vi "Periodic Tasks.vi"(8 "error in":errorcluster) -> ()   [LabVIEW 2020]
doc: "This VI runs in parallel to other robot code. It can contain as many user-defined periodic loops as you need. These can carry out PID or other sorts of timed response."
uses:
  <vilib>/Rock Robotics/WPI/Utilities/WPI_GetSetVariantRefNum.vi
  Robot Global Data.vi
  <vilib>/Rock Robotics/Network Tables/NT Read String.vi
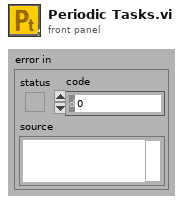
[diagram p1: front panel]
types:
  T1 = typedef "WPI_JoystickDevRef.ctl" = cluster{"Device":T2}
  T2 = typedef "WPI_JoystickDeviceEnum.ctl" = enum16{"USB 0", "USB 1", "USB 2", "USB 3", "USB 4", "USB 5"}
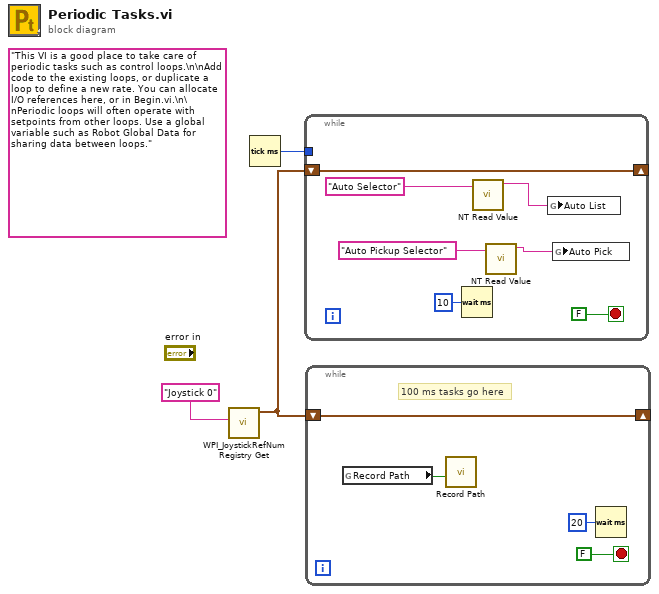
[diagram p0: block diagram]
diagram:
  (unwired) "This VI is a good place to take care of periodic tasks such as control loops.\n\nAdd code to the existing loops, or duplicate a loop to define a new rate. You can allocate I/O references here, or in Begin.vi.\n\nPeriodic loops will often operate with setpoints from other loops. Use a global variable such as Robot Global Data for sharing data between loops."
  n1 = call <vilib>:"WPI_JoystickRefNum Registry Get.vi"("refnum name"="Joystick 0") -> ("JoystickDevRef"=w2:T1)  [unwired: 1 in, 9 out]
  n2 = Tick Count (ms)() -> (millisecond timer value=w1:u32)
  n3 = while {
    shift-right: [w9] -> _
    shift-left: w2 -> [w9]
    tunnel: w1 -> [_]
    stop <- FALSE stop-if-true
    n4 = Wait (ms)(milliseconds to wait=u32 10) -> ()  [unwired: 1 out]
    n5 = call-poly <vilib>:"NT Read Value.vi"("Name"="Auto Selector") -> ("String"=w6:string)  [unwired: 9 in, 1 out]
    n6 = call-poly <vilib>:"NT Read Value.vi"("Name"="Auto Pickup Selector") -> ("String"=w7:string)  [unwired: 9 in, 1 out]
    n7 = global write "Robot Global Data.vi" "Auto List"(w6) -> ()
    n8 = global write "Robot Global Data.vi" "Auto Pick"(w7) -> ()
  }
  n9 = while {
    shift-right: [w12] -> _
    shift-left: w2 -> [w12]
    stop <- FALSE stop-if-true
    # "100 ms tasks go here"
    n10 = global read "Robot Global Data.vi" "Record Path"() -> (w11:bool)
    n11 = call "Record Path.vi"("Record Path"=w11) -> ()  [unwired: 11 in]
    n12 = Wait (ms)(milliseconds to wait=u32 20) -> ()  [unwired: 1 out]
  }
